vi "Write Line.vi"(8 "error in (no error)":errorcluster, 10 "Line":string, 11 "DigitalEffectorHardware in":refnum<class "TTLControlledDevice.lvclass">) -> (0 "error out":errorcluster, 3 "DigitalEffectorHardware out":refnum<class "TTLControlledDevice.lvclass">)   [LabVIEW 2020, in "TTLControlledDevice.lvclass"]
uses:
  TTLControlledDevice.lvclass
  TTLControlledDevice.lvclass/TTLControlledDevice.ctl
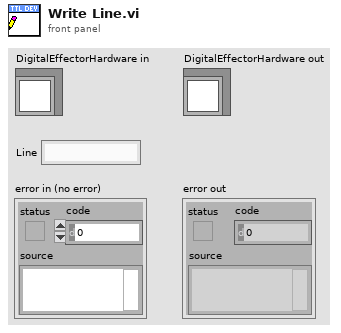
[diagram p1: front panel]
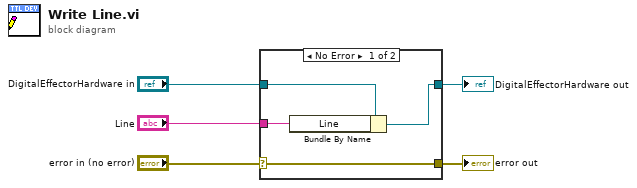
[diagram p0: block diagram]
diagram:
  n1 = case shown="No Error" "error in (no error)" {
    selector: "error in (no error)" -> [w9 w10]
    tunnel: [w9 w10] -> w4
    tunnel: [w7 w11] -> w2
    tunnel: "DigitalEffectorHardware in" -> [w8 w11]
    tunnel: "Line" -> [w6 _]
    frame No Error {
      n2 = Bundle By Name(cluster=w8, "Line"=w6) -> (w7:refnum<class "TTLControlledDevice.lvclass">)
    }
    frame Error {
    }
  }
  "error out" <- w4
  "DigitalEffectorHardware out" <- w2
